vi "#147_MAV_MSG_BATTERY_STATUS_DECODE.vi"(11 "mavlink_payload":u8[](array[numeric])) -> (3 "BATTERY_STATUS":T1)   [LabVIEW 2023]
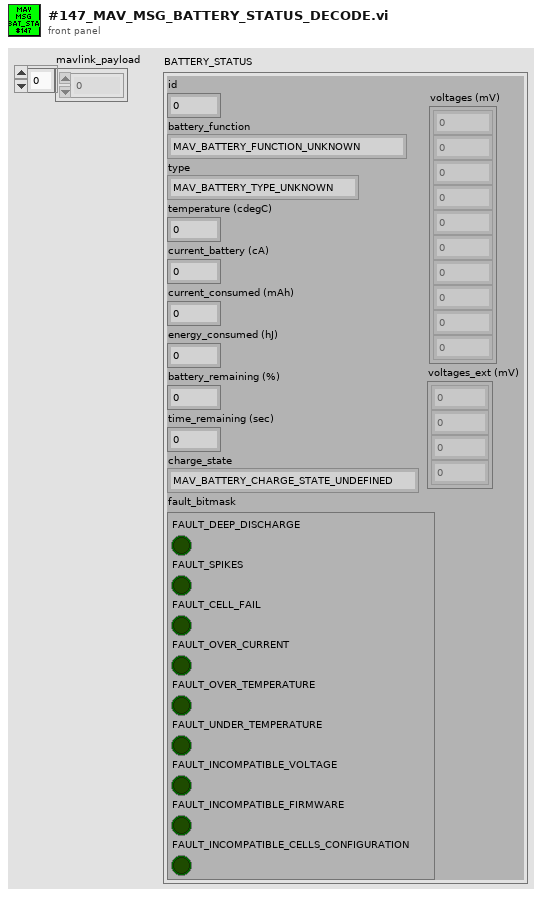
[diagram p1: front panel]
types:
  T1 = cluster{"id":u8, "battery_function":enum8{"MAV_BATTERY_FUNCTION_UNKNOWN", "MAV_BATTERY_FUNCTION_ALL", "MAV_BATTERY_FUNCTION_PROPULSION", "MAV_BATTERY_FUNCTION_AVIONICS", "MAV_BATTERY_FUNCTION_PAYLOAD"}, "type":enum8{"MAV_BATTERY_TYPE_UNKNOWN", "MAV_BATTERY_TYPE_LIPO", "MAV_BATTERY_TYPE_LIFE", "MAV_BATTERY_TYPE_LION", "MAV_BATTERY_TYPE_NIMH"}, "temperature (cdegC)":i16, "voltages (mV)":u16[], "current_battery (cA)":i16, "current_consumed (mAh)":i32, "energy_consumed (hJ)":i32, "battery_remaining (%)":i8, "time_remaining (sec)":i32, "charge_state":enum8{"MAV_BATTERY_CHARGE_STATE_UNDEFINED", "MAV_BATTERY_CHARGE_STATE_OK", "MAV_BATTERY_CHARGE_STATE_LOW", "MAV_BATTERY_CHARGE_STATE_CRITICAL", "MAV_BATTERY_CHARGE_STATE_EMERGENCY", "MAV_BATTERY_CHARGE_STATE_FAILED", "MAV_BATTERY_CHARGE_STATE_UNHEALTHY", "MAV_BATTERY_CHARGE_STATE_CHARGING"}, "voltages_ext (mV)":u16[], "fault_bitmask":cluster{"FAULT_DEEP_DISCHARGE":bool, "FAULT_SPIKES":bool, "FAULT_CELL_FAIL":bool, "FAULT_OVER_CURRENT":bool, "FAULT_OVER_TEMPERATURE":bool, "FAULT_UNDER_TEMPERATURE":bool, "FAULT_INCOMPATIBLE_VOLTAGE":bool, "FAULT_INCOMPATIBLE_FIRMWARE":bool, "FAULT_INCOMPATIBLE_CELLS_CONFIGURATION":bool}}
  T2 = enum8{"MAV_BATTERY_CHARGE_STATE_UNDEFINED", "MAV_BATTERY_CHARGE_STATE_OK", "MAV_BATTERY_CHARGE_STATE_LOW", "MAV_BATTERY_CHARGE_STATE_CRITICAL", "MAV_BATTERY_CHARGE_STATE_EMERGENCY", "MAV_BATTERY_CHARGE_STATE_FAILED", "MAV_BATTERY_CHARGE_STATE_UNHEALTHY", "MAV_BATTERY_CHARGE_STATE_CHARGING"}
  T3 = enum8{"MAV_BATTERY_TYPE_UNKNOWN", "MAV_BATTERY_TYPE_LIPO", "MAV_BATTERY_TYPE_LIFE", "MAV_BATTERY_TYPE_LION", "MAV_BATTERY_TYPE_NIMH"}
  T4 = enum8{"MAV_BATTERY_FUNCTION_UNKNOWN", "MAV_BATTERY_FUNCTION_ALL", "MAV_BATTERY_FUNCTION_PROPULSION", "MAV_BATTERY_FUNCTION_AVIONICS", "MAV_BATTERY_FUNCTION_PAYLOAD"}
  T5 = cluster{"Boolean array[0]":bool, "Boolean array[1]":bool, "Boolean array[2]":bool, "Boolean array[3]":bool, "Boolean array[4]":bool, "Boolean array[5]":bool, "Boolean array[6]":bool, "Boolean array[7]":bool, "Boolean array[8]":bool}
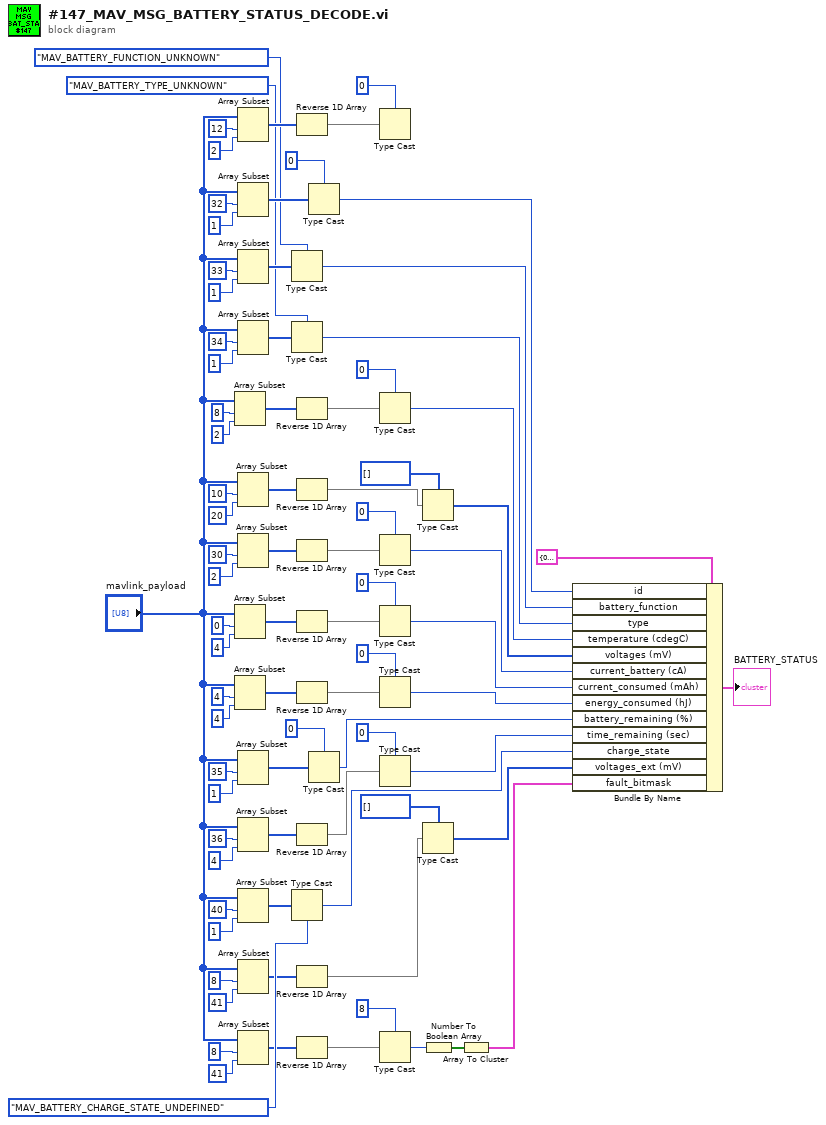
[diagram p0: block diagram]
diagram:
  n1 = Array Subset(array="mavlink_payload", index=8, length=2) -> (w61:u8[])
  n2 = Array Subset(array="mavlink_payload", index=0, length=4) -> (w49:u8[])
  n3 = Array Subset(array="mavlink_payload", index=4, length=4) -> (w43:u8[])
  n4 = Array Subset(array="mavlink_payload", index=12, length=2) -> (w79:u8[])
  n5 = Array Subset(array="mavlink_payload", index=32, length=1) -> (w75:u8[])
  n6 = Array Subset(array="mavlink_payload", index=33, length=1) -> (w71:u8[])
  n7 = Array Subset(array="mavlink_payload", index=34, length=1) -> (w66:u8[])
  n8 = Array Subset(array="mavlink_payload", index=10, length=20) -> (w54:u8[])
  n9 = Array Subset(array="mavlink_payload", index=30, length=2) -> (w15:u8[])
  n10 = Array Subset(array="mavlink_payload", index=35, length=1) -> (w36:u8[])
  n11 = Array Subset(array="mavlink_payload", index=36, length=4) -> (w32:u8[])
  n12 = Array Subset(array="mavlink_payload", index=40, length=1) -> (w26:u8[])
  n13 = Array Subset(array="mavlink_payload", index=8, length=41) -> (w21:u8[])
  n14 = Array Subset(array="mavlink_payload", index=8, length=41) -> (w5:u8[])
  n15 = Type Cast(type=T4."MAV_BATTERY_FUNCTION_UNKNOWN" ("battery_function"), x=w71) -> (*(type *) &x=w69:T4)
  n16 = Type Cast(type=T3."MAV_BATTERY_TYPE_UNKNOWN", x=w66) -> (*(type *) &x=w64:T3)
  n17 = Type Cast(type=T2."MAV_BATTERY_CHARGE_STATE_UNDEFINED" ("charge_state"), x=w26) -> (*(type *) &x=w25:T2)
  n18 = Reverse 1D Array(array=w79) -> (reversed array=w81:u8[])
  n19 = Reverse 1D Array(array=w61) -> (reversed array=w60:u8[])
  n20 = Reverse 1D Array(array=w54) -> (reversed array=w53:u8[])
  n21 = Reverse 1D Array(array=w15) -> (reversed array=w14:u8[])
  n22 = Reverse 1D Array(array=w49) -> (reversed array=w48:u8[])
  n23 = Reverse 1D Array(array=w43) -> (reversed array=w42:u8[])
  n24 = Reverse 1D Array(array=w32) -> (reversed array=w31:u8[])
  n25 = Reverse 1D Array(array=w21) -> (reversed array=w19:u8[])
  n26 = Reverse 1D Array(array=w5) -> (reversed array=w4:u8[])
  n27 = Type Cast(type=u8 0, x=w75) -> (*(type *) &x=w74:u8)
  n28 = Type Cast(type=i8 0, x=w36) -> (*(type *) &x=w35:i8)
  n29 = Type Cast(type=u16 0, x=w81) -> ()  [unwired: 1 out]
  n30 = Type Cast(type=i16 0, x=w60) -> (*(type *) &x=w58:i16)
  n31 = Type Cast(type=i16 0, x=w14) -> (*(type *) &x=w12:i16)
  n32 = Type Cast(type=0, x=w48) -> (*(type *) &x=w46:i32)
  n33 = Type Cast(type=0, x=w42) -> (*(type *) &x=w40:i32)
  n34 = Type Cast(type=0, x=w31) -> (*(type *) &x=w29:i32)
  n35 = Type Cast(type=u32 8 ("index"), x=w4) -> (*(type *) &x=w3:u32)
  n36 = Type Cast(type=u16[] [], x=w53) -> (*(type *) &x=w52:u16[])
  n37 = Type Cast(type=u16[] [], x=w19) -> (*(type *) &x=w18:u16[])
  n38 = Number To Boolean Array(number=w3) -> (Boolean array=w6:bool[])
  n39 = Array To Cluster(array=w6) -> (cluster=w1:T5)
  n40 = Bundle By Name(cluster=T1 {"id"=0, "battery_function"=enum."MAV_BATTERY_FUNCTION_UNKNOWN", "type"=enum."MAV_BATTERY_TYPE_UNKNOWN", "temperature (cdegC)"=0, "voltages (mV)"=[], "current_battery (cA)"=0, "current_consumed (mAh)"=0, "energy_consumed (hJ)"=0, "battery_remaining (%)"=0, "time_remaining (sec)"=0, "charge_state"=enum."MAV_BATTERY_CHARGE_STATE_UNDEFINED", "voltages_ext (mV)"=[], "fault_bitmask"={"FAULT_DEEP_DISCHARGE"=FALSE, "FAULT_SPIKES"=FALSE, "FAULT_CELL_FAIL"=FALSE, "FAULT_OVER_CURRENT"=FALSE, "FAULT_OVER_TEMPERATURE"=FALSE, "FAULT_UNDER_TEMPERATURE"=FALSE, "FAULT_INCOMPATIBLE_VOLTAGE"=FALSE, "FAULT_INCOMPATIBLE_FIRMWARE"=FALSE, "FAULT_INCOMPATIBLE_CELLS_CONFIGURATION"=FALSE}} ("BATTERY_STATUS"), "id"=w74, "battery_function"=w69, "type"=w64, "temperature (cdegC)"=w58, "voltages (mV)"=w52, "current_battery (cA)"=w12, "current_consumed (mAh)"=w46, "energy_consumed (hJ)"=w40, "battery_remaining (%)"=w35, "time_remaining (sec)"=w29, "charge_state"=w25, "voltages_ext (mV)"=w18, "fault_bitmask"=w1) -> (→"BATTERY_STATUS":T1)
